vi "Label Retro Targets.vi"(8 "Score Threshold":dbl=75.0, 9 "Annotate":bool=TRUE, 10 "Scores":T2(array[cluster]), 11 "Image in":T1) -> (3 "Image out":T1)   [LabVIEW 2014]
doc: "Draw text scores near or on the particle. Scores above the threshold are green and underlined."
uses:
  <vilib>/vision/Image Controls.llb/IMAQ Image.ctl
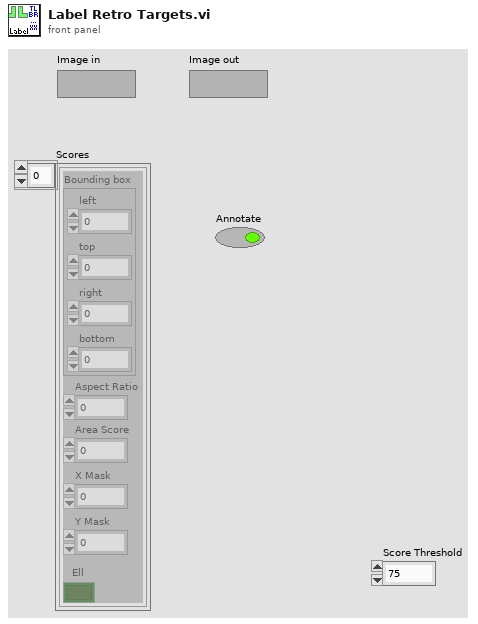
[diagram p1: front panel]
types:
  T1 = typedef "IMAQ Image.ctl" = refnum<image>
  T2 = cluster{"Bounding box":cluster{"left":dbl, "top":dbl, "right":dbl, "bottom":dbl}, "Aspect Ratio":dbl, "Area Score":dbl, "X Mask":dbl, "Y Mask":dbl, "Ell":bool}[]
  T3 = cluster{"Desired Font (Application)":enum16{"User-specified Font", "Application Font", "System Font", "Dialog Font"}, "[User-specified Font]":cluster{"Font Name":string, "Size":i16, "Strikeout?":bool, "Italic?":bool, "Underline?":bool, "Outline?":bool, "Shadow?":bool, "Bold?":bool, "Rotation Angle":dbl}, "Horizontal Alignment":i16, "Vertical Alignment":i16}
  T4 = cluster{"left":dbl, "top":dbl, "right":dbl, "bottom":dbl}
  T5 = cluster{"Aspect Ratio":dbl, "Area Score":dbl, "X Mask":dbl, "Y Mask":dbl}
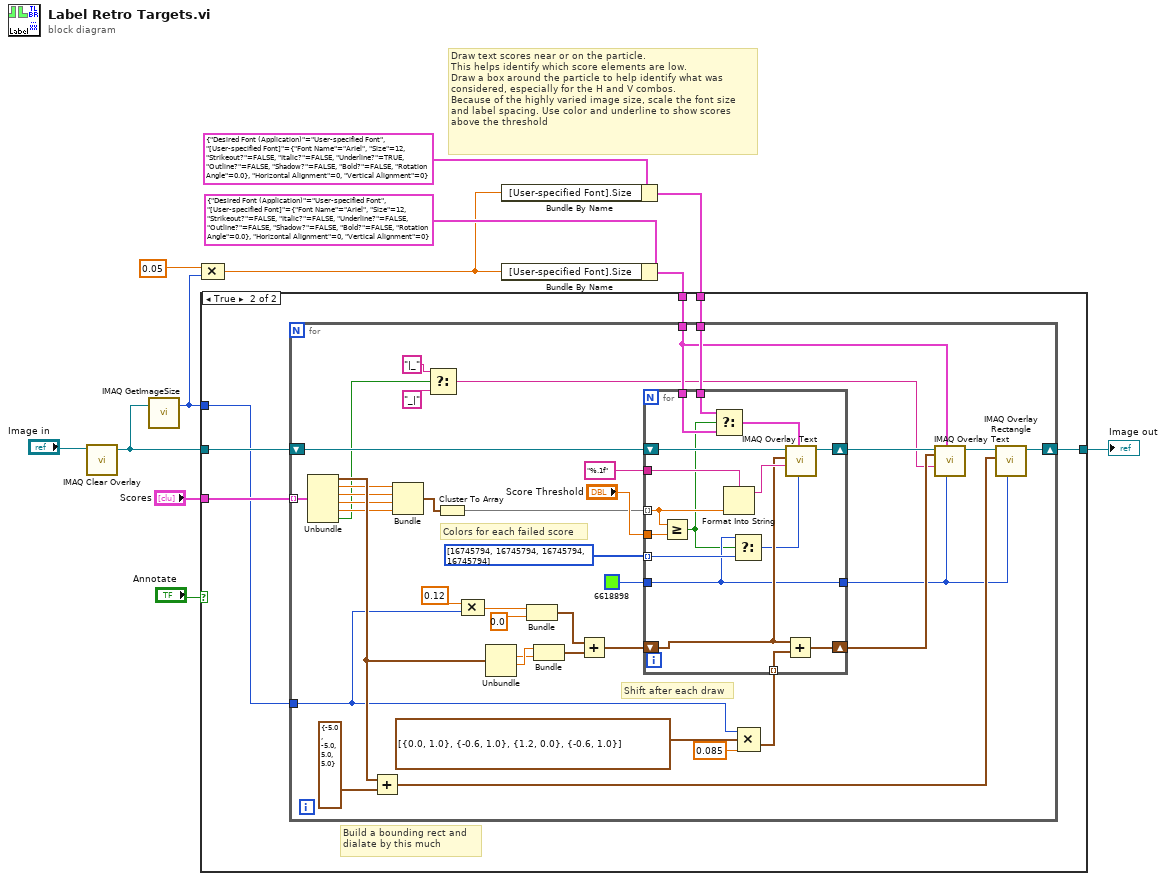
[diagram p0: block diagram]
diagram:
  # "Draw text scores near or on the particle.\nThis helps identify which score elements are low.\nDraw a box around the particle to help identify what was\nconsidered, especially for the H and V combos.\nBecause of the highly varied image size, scale the font size\nand label spacing. Use color and underline to show scores\nabove the threshold"
  n1 = call "IMAQ Clear Overlay"("Image"="Image in") -> ("Image Out"=w5:T1)  [unwired: 2 in, 8 out]
  n2 = call "IMAQ GetImageSize"("Image"=w5) -> ("Y Resolution"=w4:i32)  [unwired: 3 in, 2 out]
  n3 = Compound Arithmetic op=MULTIPLY(0.05, w4) -> (w3:dbl)
  n4 = Bundle By Name(cluster=T3 {"Desired Font (Application)"=enum."User-specified Font", "[User-specified Font]"={"Font Name"="Ariel", "Size"=12, "Strikeout?"=FALSE, "Italic?"=FALSE, "Underline?"=TRUE, "Outline?"=FALSE, "Shadow?"=FALSE, "Bold?"=FALSE, "Rotation Angle"=0.0}, "Horizontal Alignment"=0, "Vertical Alignment"=0} ("Font, Size & Style"), "[User-specified Font].Size"=w3) -> (w6:T3)
  n5 = Bundle By Name(cluster=T3 {"Desired Font (Application)"=enum."User-specified Font", "[User-specified Font]"={"Font Name"="Ariel", "Size"=12, "Strikeout?"=FALSE, "Italic?"=FALSE, "Underline?"=FALSE, "Outline?"=FALSE, "Shadow?"=FALSE, "Bold?"=FALSE, "Rotation Angle"=0.0}, "Horizontal Alignment"=0, "Vertical Alignment"=0} ("Font, Size & Style"), "[User-specified Font].Size"=w3) -> (w1:T3)
  n6 = case shown="True" "Annotate" {
    tunnel: [w13 w19] -> w12
    tunnel: "Scores" -> [_ w18]
    tunnel: w5 -> [w13 w17]
    tunnel: w6 -> [_ w16]
    tunnel: w1 -> [_ w15]
    tunnel: w4 -> [_ w14]
    frame False {
    }
    frame True {
      # "Build a bounding rect and\ndialate by this much"
      n7 = for {
        tunnel: w18 -> [w52] mode=indexing
        shift-right: [w53] -> w19
        shift-left: w17 -> [w57]
        tunnel: w14 -> [w30]
        tunnel: w16 -> [w34]
        tunnel: w15 -> [w26]
        # "Colors for each failed score"
        # "Shift after each draw"
        n8 = Unbundle(w52) -> ("Bounding box"=w46:T4, "Aspect Ratio"=w44:dbl, "Area Score"=w43:dbl, "X Mask"=w41:dbl, "Y Mask"=w42:dbl, "Ell"=w20:bool)
        n9 = Add(x=w46, y=cluster{dbl, dbl, dbl, dbl} {-5.0, -5.0, 5.0, 5.0} ("output cluster")) -> (x+y=w48:cluster{dbl, dbl, dbl, dbl})
        n10 = Bundle("Aspect Ratio"=w44, "Area Score"=w43, "X Mask"=w41, "Y Mask"=w42) -> (w54:T5)  [unwired: 1 in]
        n11 = Select(t="|_", s=w20, f="_|") -> (s? t:f=w21:string)
        n12 = Cluster To Array(cluster=w54) -> (array=w45:dbl[])
        n13 = Compound Arithmetic op=MULTIPLY(0.12, w30) -> (w31:dbl)
        n14 = Unbundle(w46) -> ("top"=w50:dbl, "right"=w51:dbl)  [unwired: 2 out]
        n15 = Bundle(w31, 0.0) -> (w33:cluster{dbl, dbl})  [unwired: 1 in]
        n16 = Bundle("right"=w51, "top"=w50) -> (w49:cluster{"right":dbl, "top":dbl})  [unwired: 1 in]
        n17 = Add(x=w33, y=w49) -> (x+y=w56:cluster{dbl, dbl})
        n18 = Compound Arithmetic op=MULTIPLY(w30, cluster{dbl, dbl}[] [{0.0, 1.0}, {-0.6, 1.0}, {1.2, 0.0}, {-0.6, 1.0}], 0.085) -> (w38:cluster{dbl, dbl}[])
        n19 = for {
          tunnel: w45 -> [w67] mode=indexing
          shift-right: [w70] -> w25
          shift-left: w56 -> [w69]
          shift-right: [w71] -> w27
          shift-left: w57 -> [w72]
          tunnel: u32[] [16745794, 16745794, 16745794, 16745794] -> [w68] mode=indexing
          tunnel: "Score Threshold" -> [w66]
          tunnel: w38 -> [w64] mode=indexing
          tunnel: "%.1f" ("format string") -> [w63]
          tunnel: u32 6618898 ("Color") -> [w62]
          tunnel: [w62] -> w24
          tunnel: w34 -> [w61]
          tunnel: w26 -> [w60]
          n20 = Greater Or Equal?(x=w67, y=w66) -> (x >= y?=w59:bool)
          n21 = Select(t=w61, s=w59, f=w60) -> (s? t:f=w58:T3)
          n22 = Format Into String(format string=w63, w67) -> (resulting string=w73:string)  [unwired: 2 in, 1 out]
          n23 = Select(t=w62, s=w59, f=w68) -> (s? t:f=w65:u32)
          n24 = Add(x=w64, y=w69) -> (x+y=w70:cluster{dbl, dbl})
          n25 = call "IMAQ Overlay Text"("Text Color (black)"=w65, "Font, Size & Style"=w58, "String"=w73, "Origin"=w69, "Image"=w72) -> ("Image Out"=w71:T1)  [unwired: 5 in, 1 out]
        }
        n26 = call "IMAQ Overlay Text"("Text Color (black)"=w24, "Font, Size & Style"=w26, "String"=w21, "Origin"=w25, "Image"=w27) -> ("Image Out"=w28:T1)  [unwired: 5 in, 1 out]
        n27 = call "IMAQ Overlay Rectangle"("Color"=w24, "Rectangle"=w48, "Image"=w28) -> ("Image Out"=w53:T1)  [unwired: 7 in, 1 out]
      }
    }
  }
  "Image out" <- w12
